vi "PID Calculation.vi"(8 "error in (no error)":errorcluster, 9 "PV":dbl, 10 "SP":dbl, 11 "PID - Data In":T1) -> (0 "error out":errorcluster, 2 "output":dbl, 3 "PID - Data Out":T1)   [LabVIEW 2024, in "cRIO1.lvlib"]
doc: "Calculates the simulation data."
uses:
  cRIO1.lvlib
  PID - Data.ctl
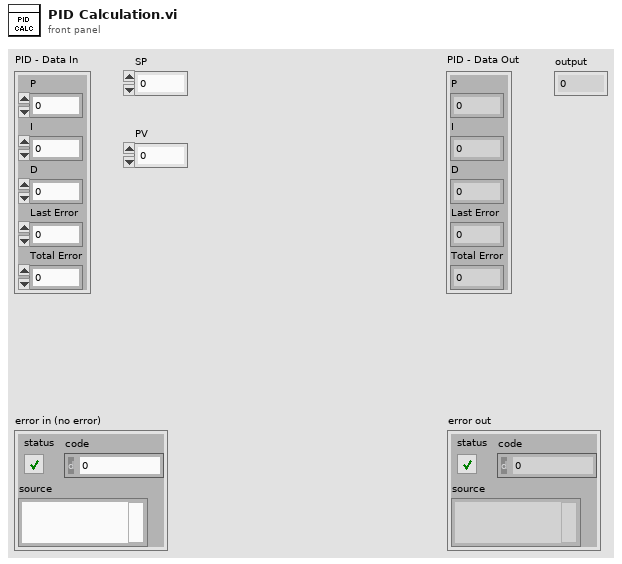
[diagram p1: front panel]
types:
  T1 = typedef "cRIO1.lvlib/PID - Data.ctl" = cluster{"P":dbl, "I":dbl, "D":dbl, "Last Error":dbl, "Total Error":dbl}
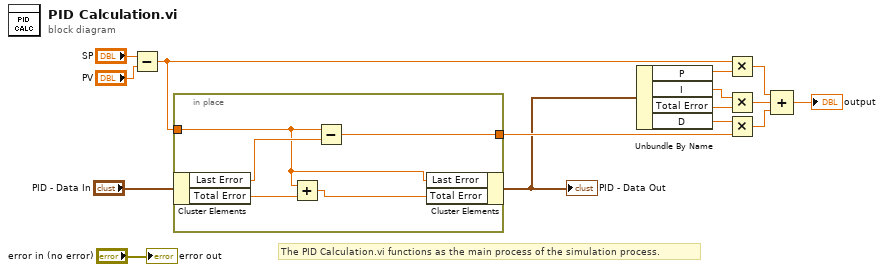
[diagram p0: block diagram]
diagram:
  # "The PID Calculation.vi functions as the main process of the simulation process."
  n1 = Subtract(x="SP", y="PV") -> (x-y=w3:dbl)
  n2 = in-place {
    in-place-border: w3 -> [w16]
    in-place-border: [w19] -> w2
    n3 = in-place-cluster #1("PID - Data In") -> ("Last Error"=w20:dbl, "Total Error"=w18:dbl)
    n4 = Add(x=w16, y=w18) -> (x+y=w17:dbl)
    n5 = Subtract(x=w16, y=w20) -> (x-y=w19:dbl)
    n6 = in-place-cluster #1("Last Error"=w16, "Total Error"=w17) -> (w1:T1)
  }
  "PID - Data Out" <- w1
  n7 = Unbundle By Name(w1) -> ("P"=w5:dbl, "I"=w12:dbl, "Total Error"=w11:dbl, "D"=w10:dbl)
  n8 = Multiply(x=w3, y=w5) -> (x*y=w9:dbl)
  n9 = Multiply(x=w12, y=w11) -> (x*y=w8:dbl)
  n10 = Multiply(x=w10, y=w2) -> (x*y=w7:dbl)
  n11 = Compound Arithmetic op=ADD(w9, w8, w7) -> (→"output":dbl)
  "error out" <- "error in (no error)"
